vi "working power measurement.vi"() -> ()   [LabVIEW 2011]
uses:
  <vilib>/DAQmx/read.llb/DAQmx Read.vi
  <vilib>/DAQmx/read.llb/DAQmx Read (Analog 1D Wfm NChan NSamp).vi
  <vilib>/DAQmx/miscellaneous.llb/DAQmx Fill In Error Info.vi
panel:
  out "data 2":waveform(dbl)[](graph) caption="data"
  out "Vde":dbl(knob) scale=0.0..5.0
  out "Vbe":dbl(knob) scale=0.0..5.0
  out "Icd":dbl(knob) scale=0.0..0.1
  out "Iab":dbl(knob) scale=0.0..0.1
  in  "Power":bool
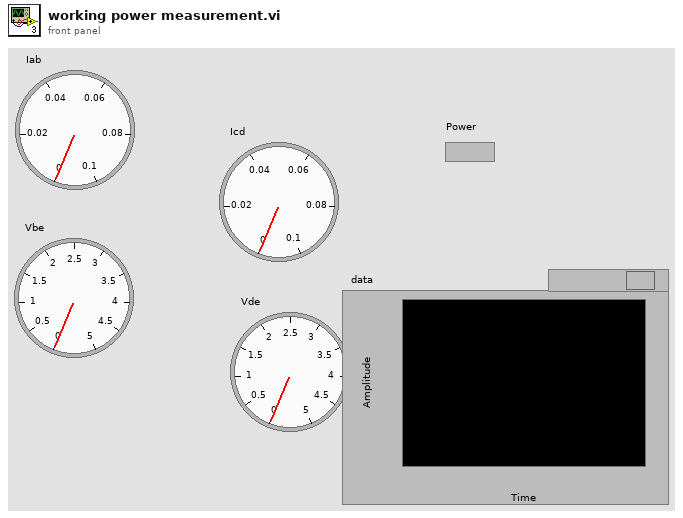
[diagram p1: front panel]
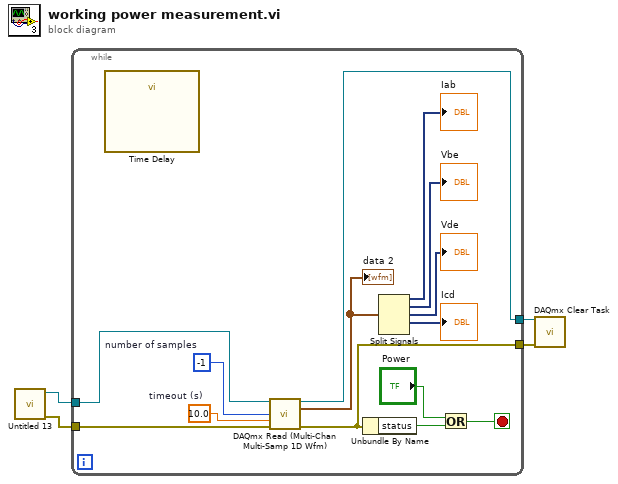
[diagram p0: block diagram]
diagram:
  n1 = call "Untitled 13.vi"() -> ("error out"=w3:errorcluster, "task out"=w4:refnum<k21>)  [unwired: 10 in]
  n2 = while {
    tunnel: w4 -> [w8]
    tunnel: w3 -> [w7]
    tunnel: [w6] -> w2
    tunnel: [w5] -> w1
    stop <- w18 stop-if-true
    w10 = 10.0  # timeout (s)
    w11 = -1  # number of samples
    n3 = call "Time Delay"() -> ()  [unwired: 11 in, 1 out]
    n4 = call-poly "DAQmx Read (Multi-Chan Multi-Samp 1D Wfm).vi"("task/channels in"=w8, "number of samples per channel"=w11, "timeout"=w10, "error in"=w7) -> ("task out"=w6:refnum<k21>, "data"=w9:waveform(dbl)[], "error out"=w5:errorcluster)  [unwired: 9 out]
    "data 2" <- w9
    n5 = Unbundle By Name(w5) -> ("status"=w16:bool)
    n6 = Split Signals(w9) -> (→"Iab":dynamicdata, →"Vbe":dynamicdata, →"Vde":dynamicdata, →"Icd":dynamicdata)  [unwired: 5 in, 1 out]
    n7 = Or(x="Power", y=w16) -> (x .or. y?=w18:bool)
  }
  n8 = call <vilib>:"DAQmx Clear Task.vi"("task in"=w2, "error in"=w1) -> ()  [unwired: 14 out]
